vi "古田污水厂流程自动启动.vi"(11 "参数":T1={"是否启用仪器"=FALSE, "CODCr"={"启动测量模式"={"测量模式"=enum."水样测量"}, "确定按钮"=TRUE}}) -> (3 "CODCr启动失败":bool)   [LabVIEW 2016, in "PLC.lvlib"]
uses:
  PLC.lvlib
  API/CodCr/CodCr.lvlib
panel:
  out "枚举":enum16{"初始化", "采配水启动", "等待", "配水", "排水", "结束"}(ring)
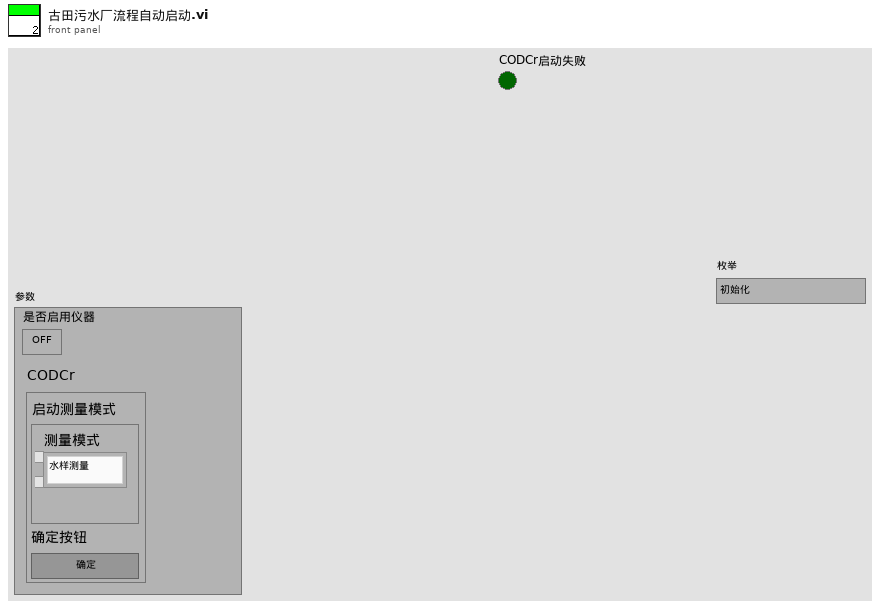
[diagram p1: front panel]
types:
  T1 = cluster{"是否启用仪器":bool, "CODCr":cluster{"启动测量模式":cluster{"测量模式":enum16{"水样测量", "标样核查", "零点核查", "加标回收", "平行样", "校零", "校标"}}, "确定按钮":bool}}
  T2 = cluster{"命令":string, cluster{"starting address":u16, "holding register value":u16}}
  T3 = enum16{"待机", "启动氨氮", "氨氮测量中", "启动总磷", "总磷测量中", "结束"}
  T4 = cluster{"测量模式":enum16{"待机", "水样测试", "标样核查", "零点核查", "跨度核查", "空白测试", "平行样测试", "加标回收", "空白校准", "标样校准", "初始化（清洗）"}, "数据标记表":string, "测量时间":dbl}
  T5 = enum16{"待机", "水样测试", "标样核查", "零点核查", "跨度核查", "空白测试", "平行样测试", "加标回收", "空白校准", "标样校准", "初始化（清洗）"}
  T6 = enum16{"空闲", "水样测试", "标样核查", "零点核查", "跨度核查", "空白测试", "平行样测试", "加标回收", "空白校准", "标样校准", "初始化（清洗）"}
  T7 = cluster{"站号":u16, "量程切换":enum32{"H", "L", "AUTO"}, "控制命令":enum16{"启动测量", "标样核查", "零点核查", "跨度核查", "空白测试", "平行样测试", "加标回收", "空白校准", "标样校准", "初始化（清洗）", "停止测试", "仪器重启", "校时", "模式设置", "测量间隔设置", "盲样测试"}, "模式设置":enum16{"待机", "连续模式", "周期模式", "定点模式", "受控模式", "手动模式"}, "测量间隔":u16}
  T8 = cluster{"时间标识":timestamp, "设备":string, "日志信息":string}
  T9 = cluster{"R0":i16, "R1":i16, "R2":i16, "R3":i16, "R4":i16, "R5":i16, "R6":i16, "R7":i16, "R8":i16, "R9":i16, "R10":i16, "R11":i16, "R12":i16, "R13":i16, "R14":i16, "R15":i16, "R16":i16, "R17":i16, "R18":i16, "R19":i16}
  T10 = enum32{"Bad", "Idle", "Run top level", "Running"}
  T11 = cluster{"测量模式":enum16{"水样测量", "标样核查", "零点核查", "加标回收", "平行样", "校零", "校标"}}
  T12 = cluster{"系统时间":timestamp, "工作状态":enum16{"空闲", "水样测试", "标样核查", "零点核查", "跨度核查", "空白测试", "平行样测试", "加标回收", "空白校准", "标样校准", "初始化（清洗）"}, "测量模式":enum16{"待机", "连续模式", "周期模式", "定点模式", "受控模式", "手动模式"}, "告警代码":enum16{"无告警", "缺试剂告警", "缺水样告警", "缺蒸馏水告警", "缺标液告警", "仪表漏液告警", "标定异常告警", "超量程告警", "加热异常", "低试剂预警", "超上限告警", "超下限告警", "仪表内部其他异常", "滴定异常告警", "电极异常告警", "量程切换告警", "参数设置告警", "PH电极电位异常", "电导率电极异常", "浊度光度异常", "溶解氧电极异常", "溶解氧光强异常", "温度异常告警", "PH异常告警", "溶解氧异常告警", "电导率异常告警", "浊度异常告警", "叶绿素异常告警", "藻密度异常告警", "蓝绿藻异常告警", "ORP异常告警", "氨氮异常告警", "清洁刷异常告警", "SD卡异常告警", "蓝牙异常告警", "Wifi异常告警", "流程异常告警"}, "故障代码":enum16{"无故障", "电机故障", "温度故障", "通讯故障", "滴定故障"}, "日志代码":u16, "软件版本":u16, "F0":sgl, "F1":sgl, "F2":sgl, "F3":sgl, "T":sgl, "H":sgl, "id":u16, "flowid":u16, "量程":u16}
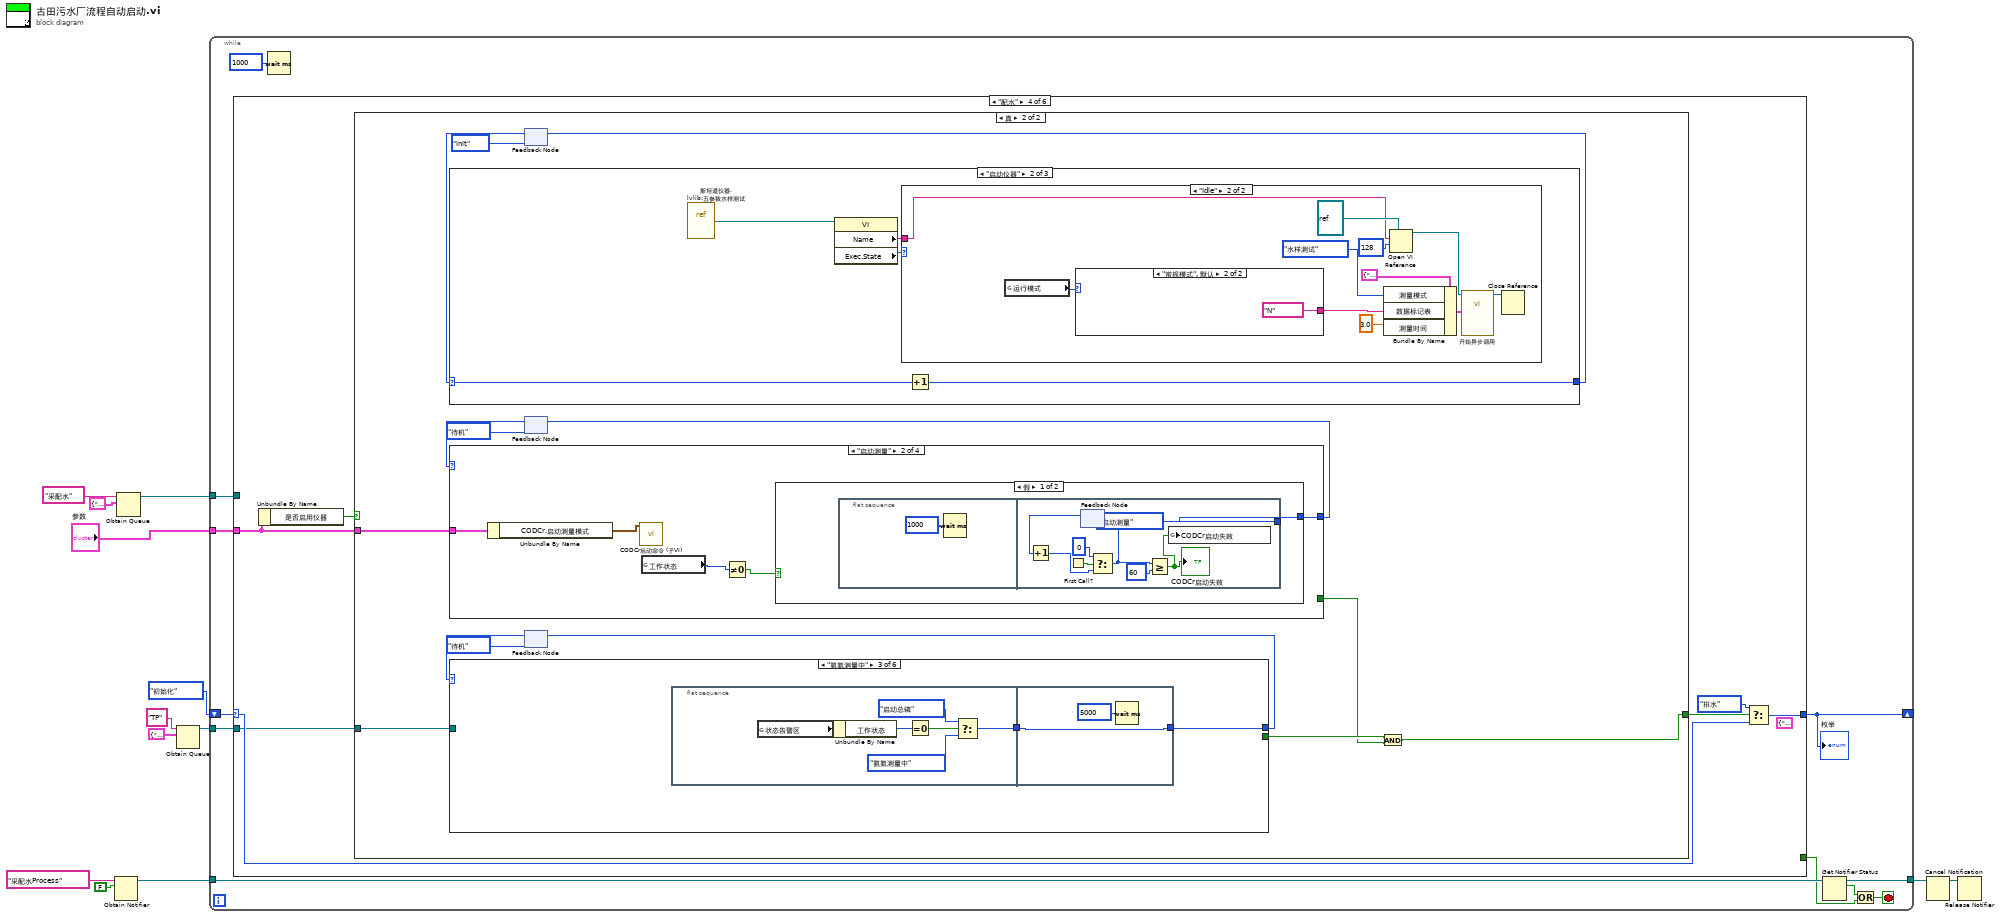
[diagram p0: block diagram]
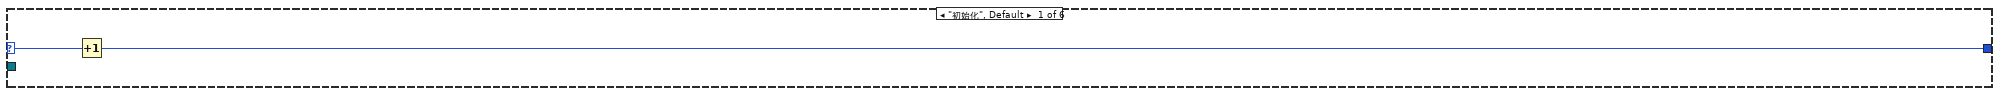
[diagram p2: hidden frame]
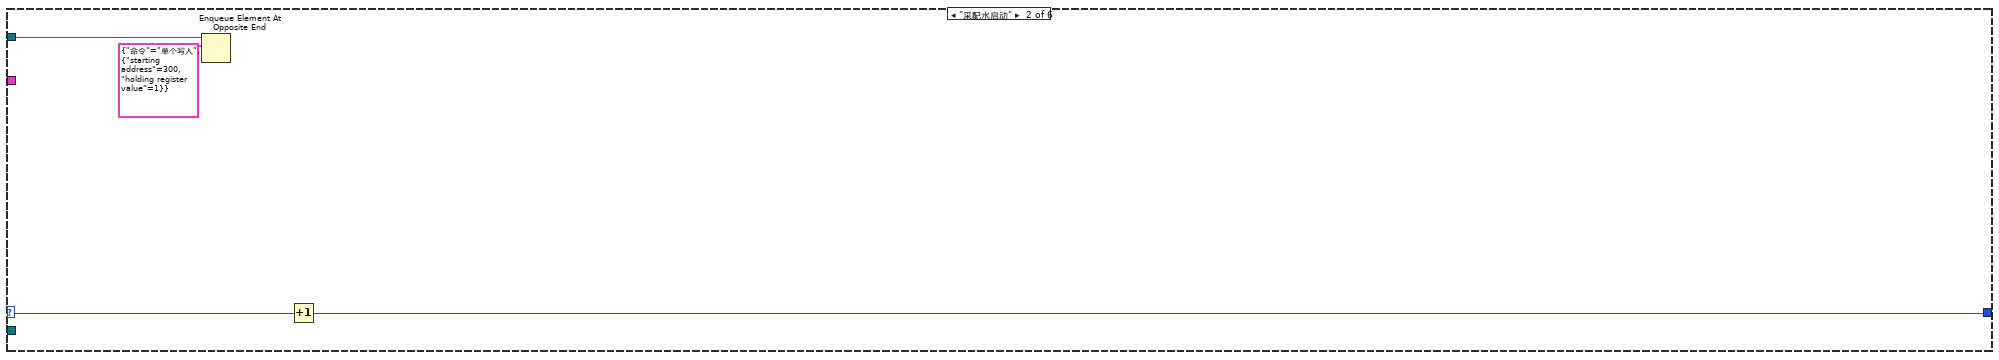
[diagram p3: hidden frame]
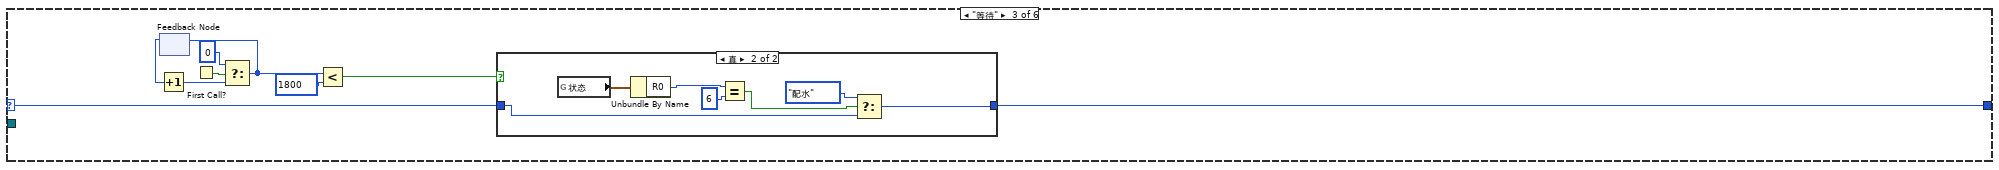
[diagram p4: hidden frame]
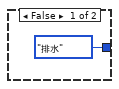
[diagram p5: hidden frame]
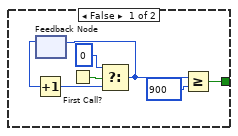
[diagram p6: hidden frame]
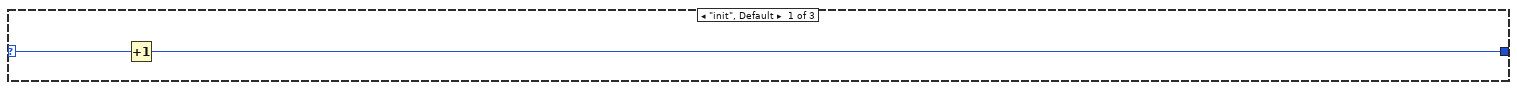
[diagram p7: hidden frame]
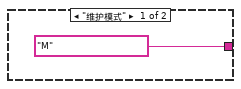
[diagram p9: hidden frame]
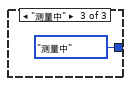
[diagram p10: hidden frame]
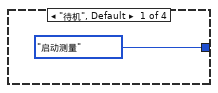
[diagram p11: hidden frame]
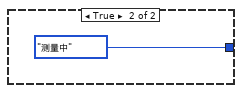
[diagram p12: hidden frame]
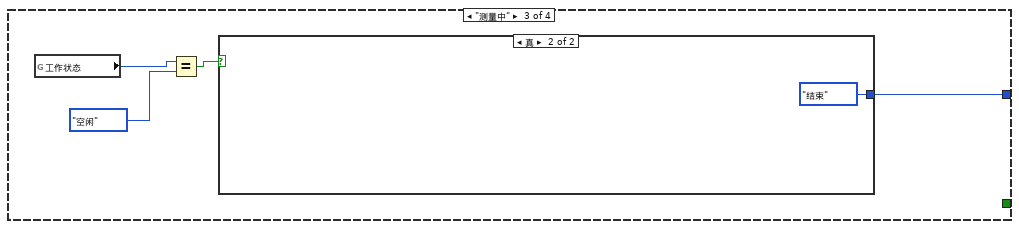
[diagram p13: hidden frame]
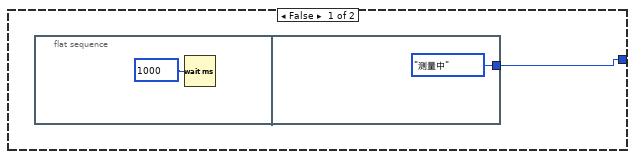
[diagram p14: hidden frame]
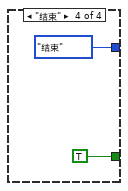
[diagram p15: hidden frame]
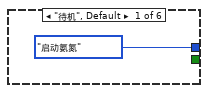
[diagram p16: hidden frame]
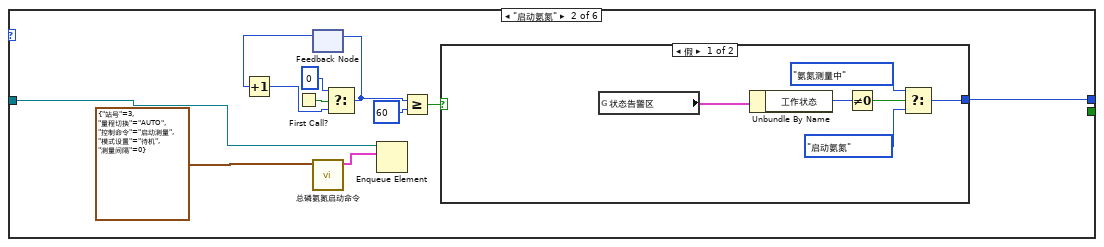
[diagram p17: hidden frame]
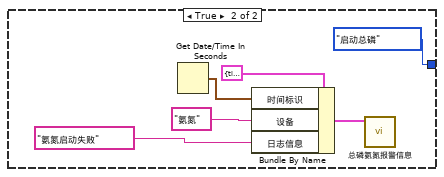
[diagram p18: hidden frame]
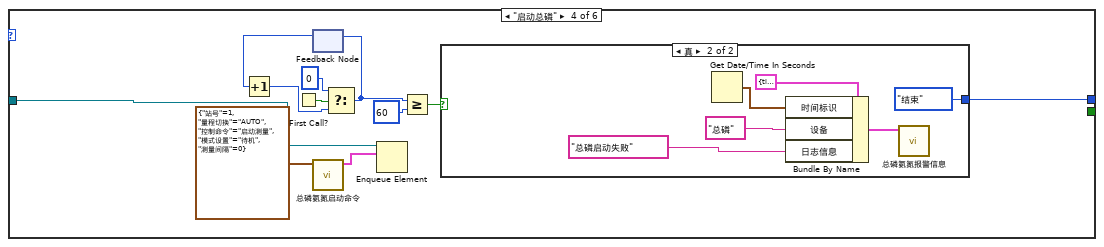
[diagram p19: hidden frame]
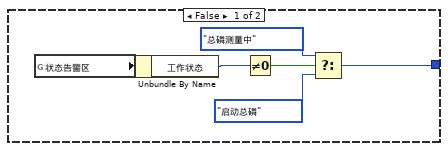
[diagram p20: hidden frame]
diagram:
  n1 = Obtain Notifier(name (unnamed)="采配水Process" ("名称（未命名）"), notification data type=FALSE) -> (notifier out=w3:refnum<notifier>)  [unwired: 2 in, 2 out]
  n2 = Obtain Queue(name (unnamed)="采配水" ("名称（未命名）"), element data type=cluster{"命令":string, "数据":variant} {"命令"="", "数据"=variant}) -> (queue out=w11:refnum<queue>)  [unwired: 3 in, 2 out]
  n3 = Obtain Queue(name (unnamed)="TP" ("名称（未命名）"), element data type=cluster{"命令":string, "data":variant} {"命令"="", "data"=variant}) -> (queue out=w7:refnum<queue>)  [unwired: 3 in, 2 out]
  n4 = while {
    tunnel: w11 -> [w24]
    shift-right: [w22] -> _
    shift-left: enum16{"初始化", "采配水启动", "等待", "配水", "排水", "结束"}."初始化" ("枚举") -> [w23]
    tunnel: w7 -> [w20]
    tunnel: "参数" -> [w19]
    tunnel: w3 -> [w18]
    tunnel: [w17] -> w2
    stop <- w16 stop-if-true
    n5 = case shown="\"配水\"" w23 {
      selector: w23 -> [w26 w28 w37 w53 w194 w199]
      tunnel: w24 -> [_ w29 _ _ w195 _]
      tunnel: [w25 w27 w36 w52 w193 w198] -> w22
      tunnel: [_ _ _ _ _ TRUE] -> w15
      tunnel: w20 -> [_ _ _ w51 _ _]
      tunnel: w19 -> [_ _ _ w48 _ _]
      frame "初始化", Default {
        n6 = Increment(x=w26) -> (x+1=w25:enum16{"初始化", "采配水启动", "等待", "配水", "排水", "结束"})
      }
      frame "采配水启动" {
        n7 = Enqueue Element At Opposite End(queue=w29, element=T2 {"命令"="单个写入", {"starting address"=300, "holding register value"=1}} ("元素")) -> ()  [unwired: 2 in, 3 out]
        n8 = Increment(x=w28) -> (x+1=w27:enum16{"初始化", "采配水启动", "等待", "配水", "排水", "结束"})
      }
      frame "等待" {
        n9 = feedback #1() -> (w33:i32)  [unwired: 1 in]
        n10 = Increment(x=w33) -> (x+1=w32:i32)
        n11 = First Call?() -> (First Call?: T/F=w34:bool)
        n12 = Select(t=0, s=w34, f=w32) -> (s? t:f=w31:i32)
        n13 = feedback-in #1(w31) -> ()
        n14 = Less?(x=w31, y=1800) -> (x < y?=w38:bool)
        n15 = case shown="真" w38 {
          tunnel: w37 -> [_ w42]
          tunnel: [enum16{"初始化", "采配水启动", "等待", "配水", "排水", "结束"}."排水" ("枚举") w41] -> w36
          frame False {
          }
          frame True {
            n16 = global read "采配水全局变量.vi" "状态"() -> (w47:T9)
            n17 = Unbundle By Name(w47) -> ("R0"=w46:i16)
            n18 = Equal?(x=w46, y=i16 6) -> (x = y?=w44:bool)
            n19 = Select(t=enum16{"初始化", "采配水启动", "等待", "配水", "排水", "结束"}."配水" ("枚举"), s=w44, f=w42) -> (s? t:f=w41:enum16{"初始化", "采配水启动", "等待", "配水", "排水", "结束"})
          }
        }
      }
      frame "配水" {
        (unwired) cluster{"命令":string, "data":variant} {"命令"="启动", "data"=variant(cluster{"站号":u16, "控制命令输出":u16[]} {"站号"=1, "控制命令输出"=[256, 0]})} ("元素")
        n20 = Unbundle By Name(w48) -> ("是否启用仪器"=w50:bool)
        n21 = case shown="真" w50 {
          tunnel: w51 -> [_ w72]
          tunnel: [w55 w62] -> w49
          tunnel: w48 -> [_ w68]
          frame False {
            n22 = feedback #2() -> (w59:i32)  [unwired: 1 in]
            n23 = Increment(x=w59) -> (x+1=w58:i32)
            n24 = First Call?() -> (First Call?: T/F=w60:bool)
            n25 = Select(t=0, s=w60, f=w58) -> (s? t:f=w56:i32)
            n26 = feedback-in #2(w56) -> ()
            n27 = Greater Or Equal?(x=w56, y=900) -> (x >= y?=w55:bool)
          }
          frame True {
            n28 = feedback #3(enum16{"init", "启动仪器", "测量中"}."init") -> (w66:enum16{"init", "启动仪器", "测量中"})
            n29 = case shown="\"启动仪器\"" w66 {
              selector: w66 -> [w77 w82 _]
              tunnel: [w76 w81 enum16{"init", "启动仪器", "测量中"}."测量中"] -> w67
              frame "init", Default {
                n30 = Increment(x=w77) -> (x+1=w76:enum16{"init", "启动仪器", "测量中"})
              }
              frame "启动仪器" {
                n31 = vi-ref "斯坦道仪器.lvlib:五参数水样测试.vi"() -> (w79:refnum<vi>)
                n32 = property class="VI"(reference=w79) -> ("Name"=w78:string, "Exec.State"=w80:T10)  [unwired: 1 in, 2 out]
                n33 = case shown="\"Idle\"" w80 {
                  tunnel: w78 -> [_ w89]
                  frame "Bad", Default {
                  }
                  frame "Idle" {
                    n34 = global read "系统变量.vi" "运行模式"() -> (w84:enum16{"维护模式", "常规模式", "应急模式", "质控模式"})
                    n35 = case shown="\"常规模式\", 默认" w84 {
                      tunnel: ["M" ("数据标记表") "N" ("数据标记表")] -> w83
                      frame "维护模式" {
                      }
                      frame "常规模式", Default {
                      }
                    }
                    n36 = Bundle By Name(cluster=T4 {"测量模式"=enum."待机", "数据标记表"="", "测量时间"=0.0} ("启动参数"), "测量模式"=T5."水样测试", "数据标记表"=w83, "测量时间"=3.0) -> (w85:T4)
                    n37 = Open VI Reference(type specifier VI Refnum (for type only)=refnum<vi> refnum ("类型说明符VI引用句柄（仅用于类型）"), vi path=w89, options=128 ("选项")) -> (vi reference=w88:refnum<vi>)  [unwired: 3 in, 1 out]
                    n38 = call-by-ref "开始异步调用"(reference=w88, "启动参数"=w85) -> (reference out=w87:refnum<vi>)  [unwired: 12 in, 1 out]
                    n39 = Close Reference(reference=w87) -> ()  [unwired: 1 in, 1 out]
                  }
                }
                n40 = Increment(x=w82) -> (x+1=w81:enum16{"init", "启动仪器", "测量中"})
              }
              frame "测量中" {
              }
            }
            n41 = feedback-in #3(w67) -> ()
            n42 = feedback #4(enum16{"待机", "启动测量", "测量中", "结束"}."待机") -> (w70:enum16{"待机", "启动测量", "测量中", "结束"})
            n43 = case shown="\"启动测量\"" w70 {
              tunnel: [enum16{"待机", "启动测量", "测量中", "结束"}."启动测量" w101 w117 enum16{"待机", "启动测量", "测量中", "结束"}."结束"] -> w69
              tunnel: w68 -> [_ w102 _ _]
              tunnel: [_ _ _ TRUE] -> w63
              frame "待机", Default {
              }
              frame "启动测量" {
                n44 = Unbundle By Name(w102) -> ("CODCr.启动测量模式"=w100:T11)
                n45 = call "CODCr启动命令 (子VI).vi"("启动测量模式"=w100) -> ()  [unwired: 11 in]
                n46 = global read "CODCr测量状态.vi" "工作状态"() -> (w99:T6)
                n47 = Not Equal To 0?(x=w99) -> (x != 0?=w98:bool)
                n48 = case shown="假" w98 {
                  tunnel: [w103 enum16{"待机", "启动测量", "测量中", "结束"}."测量中"] -> w101
                  frame False {
                    n49 = flat-sequence {
                      tunnel: [enum16{"待机", "启动测量", "测量中", "结束"}."启动测量"] -> w103
                      frame #0 {
                        n50 = Wait (ms)(milliseconds to wait=u32 1000 ("等待时间（毫秒）")) -> ()  [unwired: 1 out]
                      }
                      frame #1 {
                        n51 = First Call?() -> (First Call?: T/F=w110:bool)
                        n52 = feedback #5() -> (w109:i32)  [unwired: 1 in]
                        n53 = Increment(x=w109) -> (x+1=w108:i32)
                        n54 = Select(t=0, s=w110, f=w108) -> (s? t:f=w107:i32)
                        n55 = feedback-in #5(w107) -> ()
                        n56 = Greater Or Equal?(x=w107, y=60) -> (x >= y?=w105:bool)
                        "CODCr启动失败" <- w105
                        n57 = global write "系统变量.vi" "CODCr启动失败"(w105) -> ()
                      }
                    }
                  }
                  frame True {
                  }
                }
              }
              frame "测量中" {
                n58 = global read "CODCr测量状态.vi" "工作状态"() -> (w116:T6)
                n59 = Equal?(x=w116, y=T6."空闲" ("工作状态")) -> (x = y?=w115:bool)
                n60 = case shown="真" w115 {
                  tunnel: [w118 enum16{"待机", "启动测量", "测量中", "结束"}."结束"] -> w117
                  frame False {
                    n61 = flat-sequence {
                      tunnel: [enum16{"待机", "启动测量", "测量中", "结束"}."测量中"] -> w118
                      frame #0 {
                        n62 = Wait (ms)(milliseconds to wait=u32 1000 ("等待时间（毫秒）")) -> ()  [unwired: 1 out]
                      }
                      frame #1 {
                      }
                    }
                  }
                  frame True {
                  }
                }
              }
              frame "结束" {
              }
            }
            n63 = feedback-in #4(w69) -> ()
            n64 = feedback #6(T3."待机") -> (w74:T3)
            n65 = case shown="\"氨氮测量中\"" w74 {
              tunnel: [T3."启动氨氮" w134 w149 w167 w182 T3."结束"] -> w73
              tunnel: w72 -> [_ w135 _ w168 _ _]
              tunnel: [_ _ _ _ _ TRUE] -> w64
              frame "待机", Default {
              }
              frame "启动氨氮" {
                n66 = First Call?() -> (First Call?: T/F=w132:bool)
                n67 = feedback #7() -> (w131:i32)  [unwired: 1 in]
                n68 = Increment(x=w131) -> (x+1=w130:i32)
                n69 = call "总磷氨氮启动命令.vi"("参数"=T7 {"站号"=3, "量程切换"=enum."AUTO", "控制命令"=enum."启动测量", "模式设置"=enum."待机", "测量间隔"=0}) -> ("启动命令"=w126:cluster{"命令":string, "data":variant})  [unwired: 10 in]
                n70 = Select(t=0, s=w132, f=w130) -> (s? t:f=w129:i32)
                n71 = feedback-in #7(w129) -> ()
                n72 = Enqueue Element(queue=w135, element=w126) -> ()  [unwired: 2 in, 3 out]
                n73 = Greater Or Equal?(x=w129, y=60) -> (x >= y?=w127:bool)
                n74 = case shown="假" w127 {
                  tunnel: [w138 T3."启动总磷"] -> w134
                  frame False {
                    n75 = global read "VAR总磷氨氮全局变量.vi" "状态告警区"() -> (w141:T12)
                    n76 = Unbundle By Name(w141) -> ("工作状态"=w140:T6)
                    n77 = Not Equal To 0?(x=w140) -> (x != 0?=w139:bool)
                    n78 = Select(t=T3."氨氮测量中", s=w139, f=T3."启动氨氮") -> (s? t:f=w138:T3)
                  }
                  frame True {
                    n79 = Get Date/Time In Seconds() -> (seconds since 1Jan1904=w146:timestamp)
                    n80 = Bundle By Name(cluster=T8 {"时间标识"=timestamp(0 s since 1904-01-01), "设备"="", "日志信息"=""} ("data in"), "时间标识"=w146, "设备"="氨氮", "日志信息"="氨氮启动失败") -> (w142:T8)
                    n81 = call "总磷氨氮报警信息.vi"("data in"=w142) -> ()  [unwired: 11 in]
                  }
                }
              }
              frame "氨氮测量中" {
                n82 = flat-sequence {
                  tunnel: [w153] -> w148
                  tunnel: [w157] -> w149
                  tunnel: w148 -> [w157]
                  frame #0 {
                    n83 = global read "VAR总磷氨氮全局变量.vi" "状态告警区"() -> (w154:T12)
                    n84 = Unbundle By Name(w154) -> ("工作状态"=w155:T6)
                    n85 = Equal To 0?(x=w155) -> (x = 0?=w152:bool)
                    n86 = Select(t=T3."启动总磷", s=w152, f=T3."氨氮测量中") -> (s? t:f=w153:T3)
                  }
                  frame #1 {
                    n87 = Wait (ms)(milliseconds to wait=u32 5000 ("等待时间（毫秒）")) -> ()  [unwired: 1 out]
                  }
                }
              }
              frame "启动总磷" {
                n88 = First Call?() -> (First Call?: T/F=w165:bool)
                n89 = feedback #8() -> (w164:i32)  [unwired: 1 in]
                n90 = Increment(x=w164) -> (x+1=w163:i32)
                n91 = call "总磷氨氮启动命令.vi"("参数"=T7 {"站号"=1, "量程切换"=enum."AUTO", "控制命令"=enum."启动测量", "模式设置"=enum."待机", "测量间隔"=0}) -> ("启动命令"=w159:cluster{"命令":string, "data":variant})  [unwired: 10 in]
                n92 = Select(t=0, s=w165, f=w163) -> (s? t:f=w162:i32)
                n93 = feedback-in #8(w162) -> ()
                n94 = Enqueue Element(queue=w168, element=w159) -> ()  [unwired: 2 in, 3 out]
                n95 = Greater Or Equal?(x=w162, y=60) -> (x >= y?=w160:bool)
                n96 = case shown="真" w160 {
                  tunnel: [w171 T3."结束"] -> w167
                  frame False {
                    n97 = global read "VAR总磷氨氮全局变量.vi" "状态告警区"() -> (w172:T12)
                    n98 = Unbundle By Name(w172) -> ("工作状态"=w173:T6)
                    n99 = Not Equal To 0?(x=w173) -> (x != 0?=w174:bool)
                    n100 = Select(t=T3."总磷测量中", s=w174, f=T3."启动总磷") -> (s? t:f=w171:T3)
                  }
                  frame True {
                    n101 = Get Date/Time In Seconds() -> (seconds since 1Jan1904=w180:timestamp)
                    n102 = Bundle By Name(cluster=T8 {"时间标识"=timestamp(0 s since 1904-01-01), "设备"="", "日志信息"=""} ("data in"), "时间标识"=w180, "设备"="总磷", "日志信息"="总磷启动失败") -> (w175:T8)
                    n103 = call "总磷氨氮报警信息.vi"("data in"=w175) -> ()  [unwired: 11 in]
                  }
                }
              }
              frame "总磷测量中" {
                n104 = flat-sequence {
                  tunnel: [w186] -> w181
                  tunnel: [w190] -> w182
                  tunnel: w181 -> [w190]
                  frame #0 {
                    n105 = global read "VAR总磷氨氮全局变量.vi" "状态告警区"() -> (w187:T12)
                    n106 = Unbundle By Name(w187) -> ("工作状态"=w188:T6)
                    n107 = Equal To 0?(x=w188) -> (x = 0?=w185:bool)
                    n108 = Select(t=T3."结束", s=w185, f=T3."总磷测量中") -> (s? t:f=w186:T3)
                  }
                  frame #1 {
                    n109 = Wait (ms)(milliseconds to wait=u32 5000 ("等待时间（毫秒）")) -> ()  [unwired: 1 out]
                  }
                }
              }
              frame "结束" {
              }
            }
            n110 = feedback-in #6(w73) -> ()
            n111 = And(x=w64, y=w63) -> (x .and. y?=w62:bool)
          }
        }
        n112 = Select(t=enum16{"初始化", "采配水启动", "等待", "配水", "排水", "结束"}."排水" ("枚举"), s=w49, f=w53) -> (s? t:f=w52:enum16{"初始化", "采配水启动", "等待", "配水", "排水", "结束"})
      }
      frame "排水" {
        n113 = Enqueue Element At Opposite End(queue=w195, element=T2 {"命令"="单个写入", {"starting address"=303, "holding register value"=1}} ("元素")) -> ()  [unwired: 2 in, 3 out]
        n114 = Increment(x=w194) -> (x+1=w193:enum16{"初始化", "采配水启动", "等待", "配水", "排水", "结束"})
      }
      frame "结束" {
        n115 = Increment(x=w199) -> (x+1=w198:enum16{"初始化", "采配水启动", "等待", "配水", "排水", "结束"})
      }
    }
    "枚举" <- w22
    n116 = Wait (ms)(milliseconds to wait=u32 1000 ("等待时间（毫秒）")) -> ()  [unwired: 1 out]
    n117 = Get Notifier Status(notifier=w18) -> (notifier out=w17:refnum<notifier>, current notification=w14:bool)  [unwired: 1 in, 3 out]
    n118 = Or(x=w14, y=w15) -> (x .or. y?=w16:bool)
  }
  n119 = Cancel Notification(0:w2) -> (8:w1:refnum<notifier>)  [unwired: 1 in, 2 out]
  n120 = Release Notifier(notifier=w1) -> ()  [unwired: 2 in, 3 out]
